vi "SHI_Cryopump_interface.vi"() -> ()   [LabVIEW 2017]
uses:
  Type_Defs/Cryo_Pump_MCC_Status.ctl
  Type_Defs/Cryo_Pump_MCC_CryoPump.ctl
  Type_Defs/Cryo_Pump_MCC_RoughingInterlock.ctl
  Type_Defs/Cryo_Pump_MCC_Status_Status.ctl
  Type_Defs/Cryo_Pump_MCC_Start_Regen.ctl
  Type_Defs/Cryo_Pump_MCC_First_Stage_Temp_CTL.ctl
  Type_Defs/Cryo_Pump_MCC_Params_Power_Failure_Recovery.ctl
  Type_Defs/Cryo_Pump_MCC_Regen_Params.ctl
  Type_Defs/Cryo_Pump_Compressor_Status.ctl
  Type_Defs/Cryo_Pump_Compressor_Status_Status.ctl
  <vilib>/httpClient/ClientHandle.ctl
  Type_Defs/Cryo_Pump_Plots.ctl
  Type_Defs/Cryo_Pump_MCC_Params.ctl
  msg7171_linux.llb/send single message.vi
  msg7171_linux.llb/send multiple messages.vi
  <vilib>/httpClient/POSTBuffer.vi
  <vilib>/httpClient/LabVIEWHTTPClient.lvlib
panel:
  in  "Cold Head Start":bool
  in  "Compressor On":bool
  in  "Roughing_Ilock_Permission":bool
  in  "TC_Pressure_Guage":bool
  in  "Roughing Valve":bool
  in  "Purge Valve":bool
  in  "Send Regen Start":bool
  out "Compressor":T1
  in  "2nd Stage Temp CTL":u32 max=320 step=1
  out "Regen Time":u32
  out "Regen Step Timer":u32
  in  "Regen Start Delay":u32 max=59994 step=1
  in  "Regen Parameters":T3 {"z" max=1 step=1; "G" max=9999 step=1; "C" min=1 max=3 step=1; "A" max=1 step=1; "6" max=80 step=1; "5" max=200 step=1; "4" min=1 max=100 step=1; "3" min=25 max=200 step=1; "2" max=200 step=1; "1" max=9990 step=1; "0" max=59994 step=1}
  out "Regen Cycles":u32
  out "Power Failure Recovery Status":string
  in  "Power Failure Recovery":T4 items=["Disabled", "Enabled", "Enabled only when Stage 2 < Restart Temp."]
  out "MCC Version":string
  out "Last Rate Of Rise Value":u32
  in  "1st Stage Temp Ctl":T5 {"method" items=["ExtHeat", "1st s ctl", "2nd sctl", "Dual"]; "temp" max=320 step=1}
  out "Failed Repurge Cycles":u32
  out "Failed Rate Of Rise Cycles":u32
  out "Elapsed Time":u32
  in  "Start Regen Parameter":T6=enum."Start full regeneration cycle"
  out "MCC Status":T7
  out "Get Params json":string
  out "Get Status json":string
  in  "exit":bool
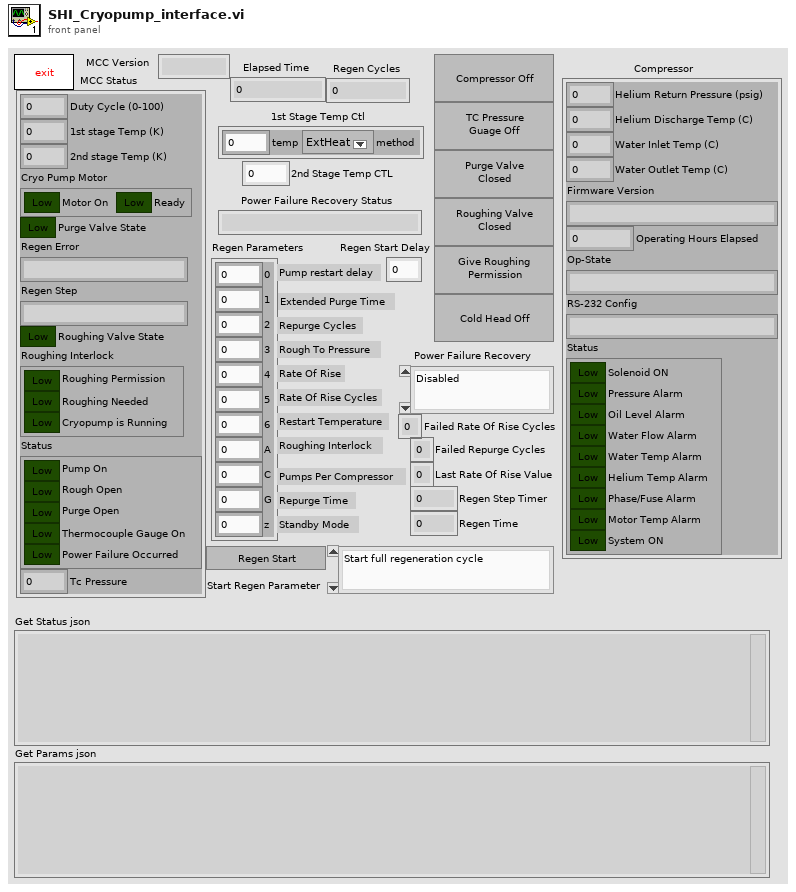
[diagram p1: front panel]
types:
  T1 = typedef "Cryo_Pump_Compressor_Status.ctl" = cluster{"Helium Return Pressure (psig)":u32, "Helium Discharge Temp (C)":u32, "Water Inlet Temp (C)":u32, "Water Outlet Temp (C)":u32, "Firmware Version":string, "Operating Hours Elapsed":dbl, "Op-State":string, "RS-232 Config":string, "Status":T2}
  T2 = typedef "Cryo_Pump_Compressor_Status_Status.ctl" = cluster{"Solenoid ON":bool, "Pressure Alarm":bool, "Oil Level Alarm":bool, "Water Flow Alarm":bool, "Water Temp Alarm":bool, "Helium Temp Alarm":bool, "Phase/Fuse Alarm":bool, "Motor Temp Alarm":bool, "System ON":bool}
  T3 = typedef "Cryo_Pump_MCC_Regen_Params.ctl" = cluster{"0":u32, "1":u32, "2":u32, "3":u32, "4":u32, "5":u32, "6":u32, "A":u32, "C":u32, "G":u32, "z":u32}
  T4 = typedef "Cryo_Pump_MCC_Params_Power_Failure_Recovery.ctl" = u16
  T5 = typedef "Cryo_Pump_MCC_First_Stage_Temp_CTL.ctl" = cluster{"temp":u32, "method":u32}
  T6 = typedef "Cryo_Pump_MCC_Start_Regen.ctl" = enum16{"Abort current regeneration cycle", "Start full regeneration cycle", "Start fast regeneration cycle", "Activate stand-by pump module for normal pumping operation", "Warm up cryopump and stop"}
  T7 = typedef "Cryo_Pump_MCC_Status.ctl" = cluster{"Duty Cycle (0-100)":dbl, "1st stage Temp (K)":dbl, "2nd stage Temp (K)":dbl, "Cryo Pump Motor":T8, "Purge Valve State":bool, "Regen Error":string, "Regen Step":string, "Roughing Valve State":bool, "Roughing Interlock":T9, "Status":T10, "Tc Pressure":dbl}
  T8 = typedef "Cryo_Pump_MCC_CryoPump.ctl" = cluster{"Motor On":bool, "Ready":bool}
  T9 = typedef "Cryo_Pump_MCC_RoughingInterlock.ctl" = cluster{"Roughing Permission":bool, "Roughing Needed":bool, "Cryopump is Running":bool}
  T10 = typedef "Cryo_Pump_MCC_Status_Status.ctl" = cluster{"Pump On":bool, "Rough Open":bool, "Purge Open":bool, "Thermocouple Gauge On":bool, "Power Failure Occurred":bool}
  T11 = typedef "Cryo_Pump_Plots.ctl" = cluster{"Duty Cycle (0-100)":dbl, "1st stage Temp (K)":dbl, "2nd stage Temp (K)":dbl, "Helium Return Pressure (psig)":u32, "Helium Discharge Temp (C)":u32, "Water Inlet Temp (C)":u32, "Water Outlet Temp (C)":u32}
  T12 = typedef "LabVIEWHTTPClient.lvlib/ClientHandle.ctl" = refnum<k1>
  T13 = cluster{"go":bool, "Http session":T12, "URL prefex":string, "Next get param":u32}
  T14 = typedef "Cryo_Pump_MCC_Params.ctl" = cluster{"MCC Version":string, "First Stage Temp CTL":T5, "Second Stage Temp CTL":u32, "Tc Pressure State":bool, "Elapsed Time":u32, "Power Failure Recovery":T4, "Power Failure Recovery Status":string, "Regen Time":u32, "Regen Parameters":T3, "Regen Start Delay":u32, "Regen Step Timer":u32, "Failed Rate Of Rise Cycles":u32, "Failed Repurge Cycles":u32, "Last Rate Of Rise Value":u32, "Regen Cycles":u32}
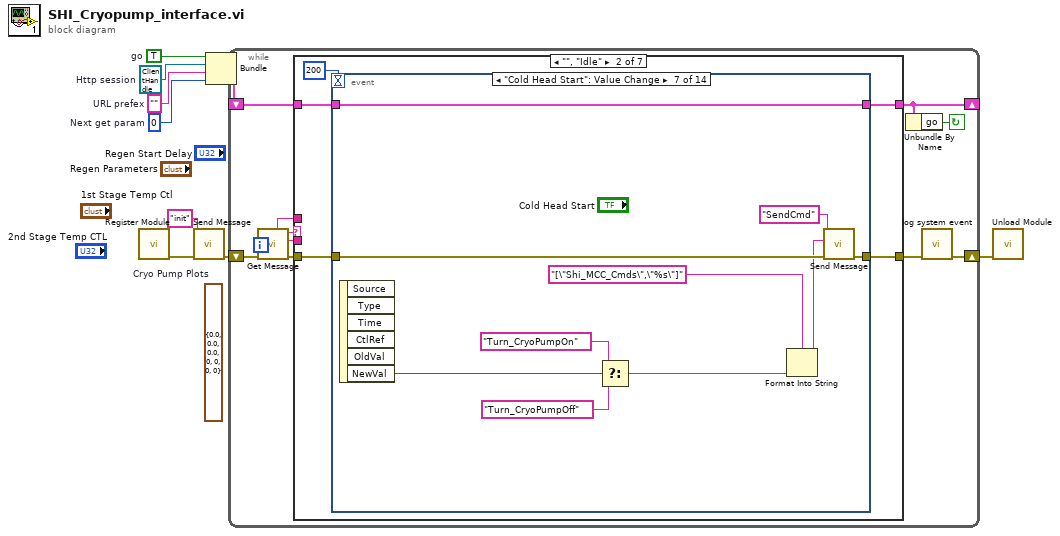
[diagram p0: block diagram]
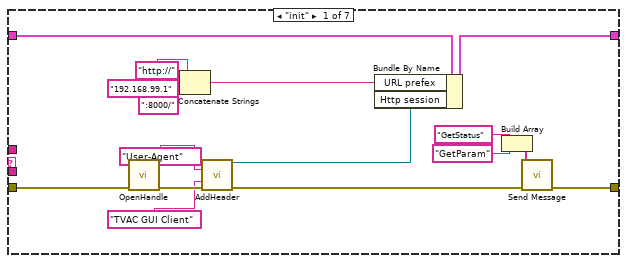
[diagram p2: hidden frame]
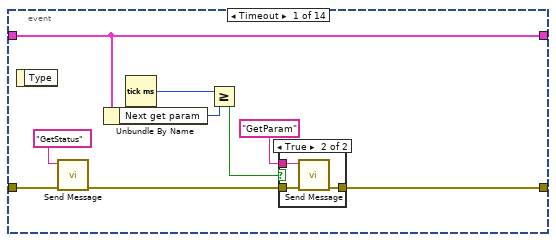
[diagram p3: hidden frame]
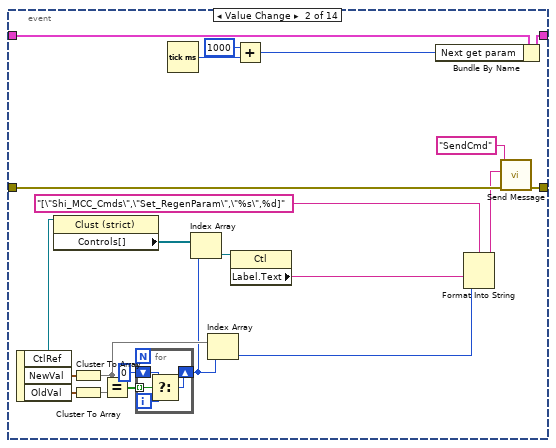
[diagram p5: hidden frame]
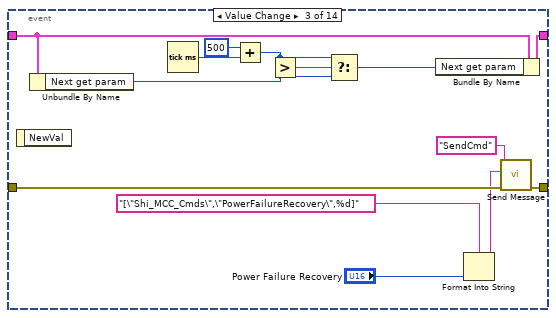
[diagram p6: hidden frame]
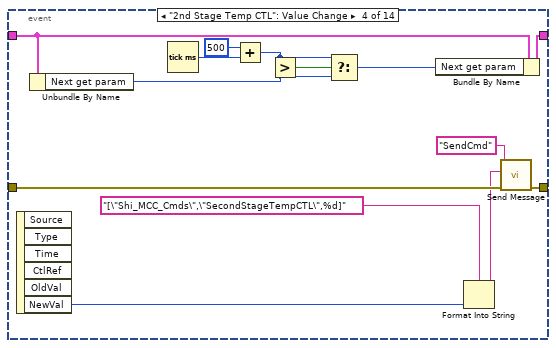
[diagram p7: hidden frame]
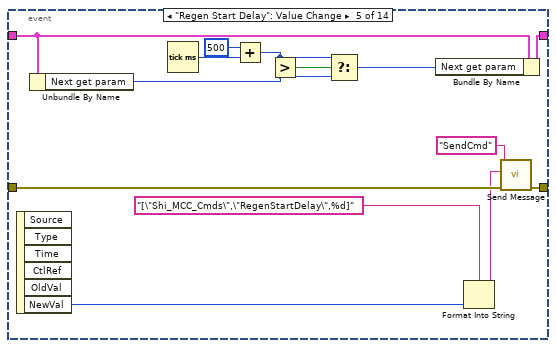
[diagram p8: hidden frame]
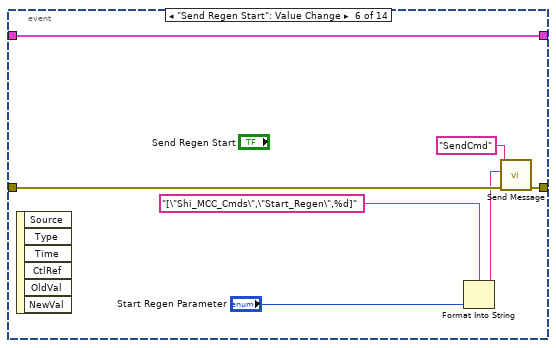
[diagram p9: hidden frame]
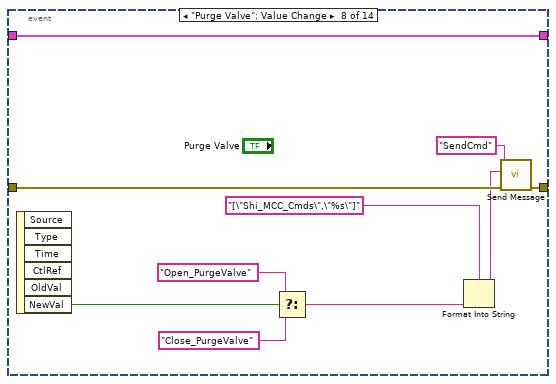
[diagram p10: hidden frame]
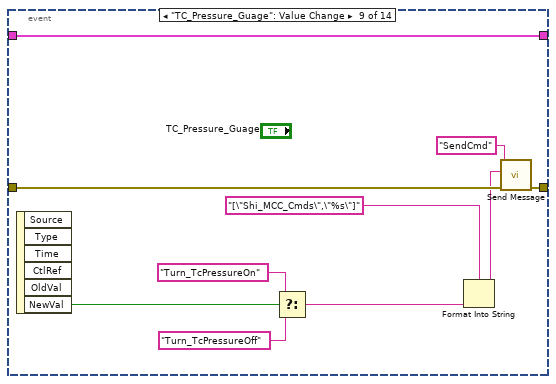
[diagram p11: hidden frame]
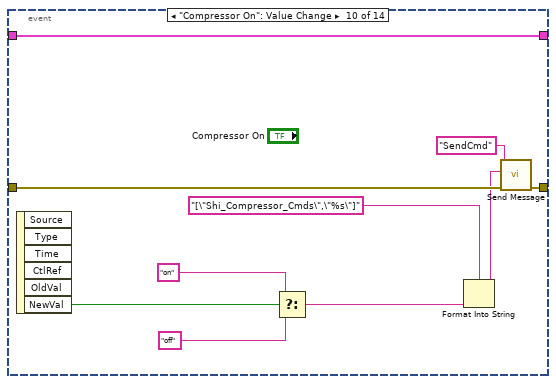
[diagram p12: hidden frame]
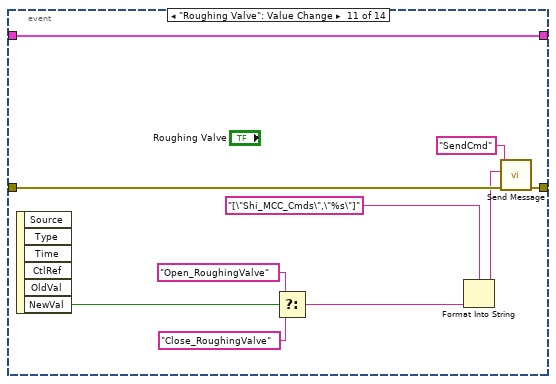
[diagram p13: hidden frame]
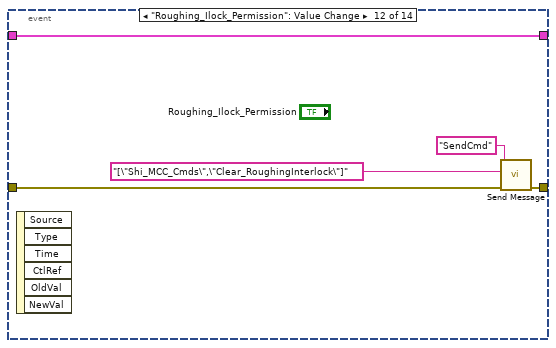
[diagram p14: hidden frame]
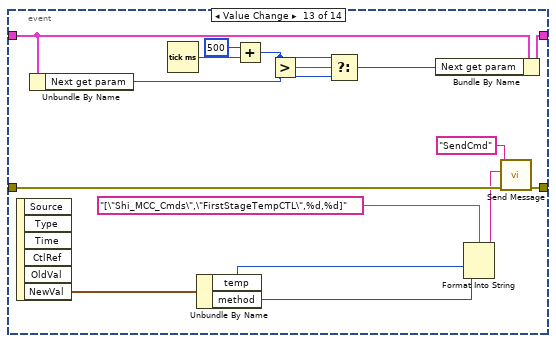
[diagram p15: hidden frame]
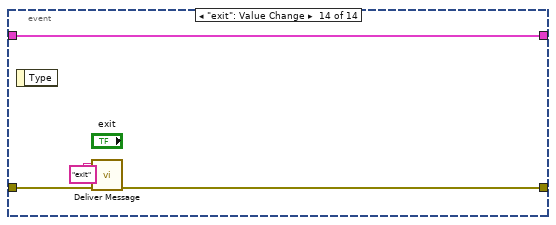
[diagram p16: hidden frame]
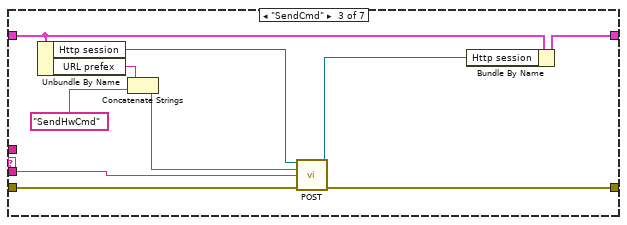
[diagram p17: hidden frame]
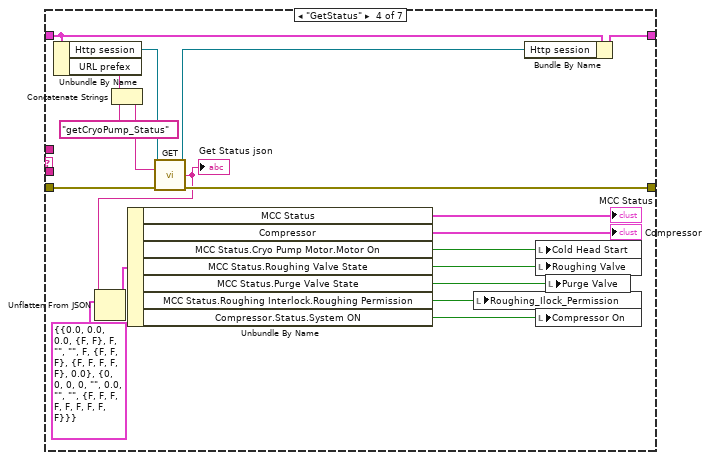
[diagram p18: hidden frame]
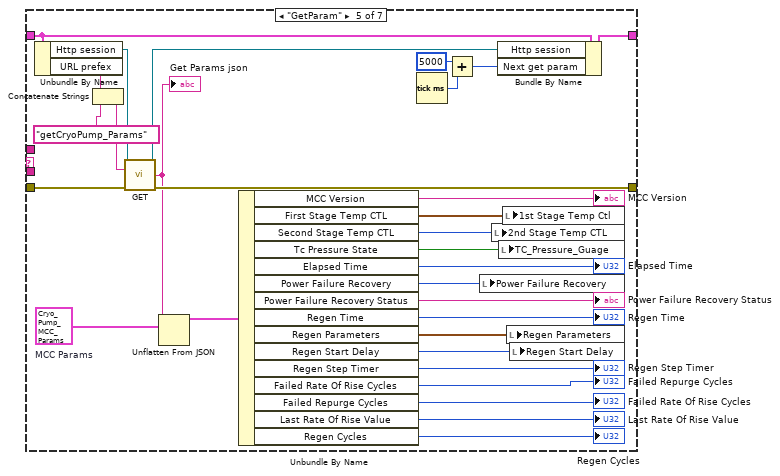
[diagram p19: hidden frame]
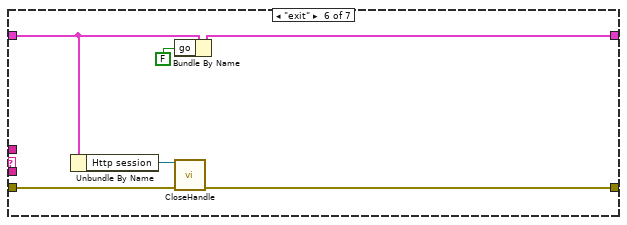
[diagram p20: hidden frame]
diagram:
  (unwired) T11 {"Duty Cycle (0-100)"=0.0, "1st stage Temp (K)"=0.0, "2nd stage Temp (K)"=0.0, "Helium Return Pressure (psig)"=0, "Helium Discharge Temp (C)"=0, "Water Inlet Temp (C)"=0, "Water Outlet Temp (C)"=0}  # Cryo Pump Plots
  w1 = u32 0  # Next get param
  w5 = ""  # URL prefex
  w6 = T12 refnum  # Http session
  w7 = TRUE  # go
  n1 = call "Register Module.vi"() -> ("error out"=w3:errorcluster)  [unwired: 10 in, 1 out]
  n2 = call-poly "Send Message.vi"("error in (no error)"=w3, "event"="init") -> ("error out"=w2:errorcluster)  [unwired: 9 in]
  n3 = Bundle("go"=w7, "Http session"=w6, "URL prefex"=w5, "Next get param"=w1) -> (w9:T13)  [unwired: 1 in]
  n4 = while {
    shift-left: w9 -> [w16]
    shift-right: [w13] -> _
    shift-right: [w11] -> w8
    shift-left: w2 -> [w19]
    stop <- w12 continue-if-true
    n5 = call "Get Message.vi"("error in (no error)"=w19) -> ("error out"=w17:errorcluster, "event buffer"=w18:string, "event"=w15:string, "source"=w14:string)  [unwired: 7 in]
    n6 = case shown="\"\", \"Idle\"" w15 {
      selector: w15 -> [_ _ _ _ _ _ w272]
      tunnel: [w27 w38 w209 w226 w256 w269 w274] -> w13
      tunnel: w16 -> [w36 w37 w208 w225 w255 w264 w274]
      tunnel: w18 -> [_ _ w205 _ _ _ _]
      tunnel: w17 -> [w31 w39 w207 w228 w258 w267 w273]
      tunnel: w14 -> [_ _ _ _ _ _ w271]
      tunnel: [w23 w41 w206 w227 w257 w266 w270] -> w10
      frame "init" {
        n7 = call <vilib>:"OpenHandle.vi"("error in (no error)"=w31) -> ("client handle out"=w32:T12, "error out"=w35:errorcluster)  [unwired: 13 in]
        n8 = Concatenate Strings("http://" ("url"), "192.168.99.1" ("Address"), ":8000/" ("url")) -> (w26:string)
        n9 = call <vilib>:"AddHeader.vi"("client handle"=w32, "header"="User-Agent", "value"="TVAC GUI Client", "error in (no error)"=w35) -> ("client handle out"=w25:T12, "error out"=w24:errorcluster)  [unwired: 10 in]
        n10 = Bundle By Name(cluster=w36, "URL prefex"=w26, "Http session"=w25) -> (w27:T13)
        n11 = Build Array("GetStatus" ("event"), "GetParam" ("event")) -> (w21:string[])
        n12 = call-poly "Send Message.vi"("error in (no error)"=w24, "event"=w21) -> ("error out"=w23:errorcluster)  [unwired: 9 in]
      }
      frame "", "Idle" {
        n13 = event shown="[6] \"Cold Head Start\": Value Change" {
          selector: _ -> [_ _ _ _ _ _ _ _ _ _ _ _ _ _]
          dyn-events: _ -> [_ _ _ _ _ _ _ _ _ _ _ _ _ _]
          timeout: 200 ("milliseconds to wait") -> [_ _ _ _ _ _ _ _ _ _ _ _ _ _]
          tunnel: w39 -> [w50 w72 w94 w108 w122 w129 w139 w149 w159 w169 w179 w184 w200 w204]
          tunnel: [w46 w71 w93 w107 w121 w128 w138 w148 w158 w168 w178 w183 w199 w203] -> w41
          tunnel: [w42 w58 w88 w102 w116 w123 w130 w140 w150 w160 w170 w180 w194 w201] -> w38
          tunnel: w37 -> [w42 w59 w89 w103 w117 w123 w130 w140 w150 w160 w170 w180 w195 w201]
          event Timeout {
            n14 = event-data() -> ()  [unwired: 1 in, 1 out]
            n15 = call-poly "Send Message.vi"("error in (no error)"=w50, "event"="GetStatus") -> ("error out"=w48:errorcluster)  [unwired: 9 in]
            n16 = Unbundle By Name(w42) -> ("Next get param"=w43:u32)
            n17 = Tick Count (ms)() -> (millisecond timer value=w45:u32)
            n18 = Greater Or Equal?(x=w45, y=w43) -> (x >= y?=w44:bool)
            n19 = case shown="True" w44 {
              tunnel: w48 -> [w51 w54]
              tunnel: [w51 w53] -> w46
              tunnel: "GetParam" ("event") -> [_ w52]
              frame False {
              }
              frame True {
                n20 = call-poly "Send Message.vi"("error in (no error)"=w54, "event"=w52) -> ("error out"=w53:errorcluster)  [unwired: 9 in]
              }
            }
          }
          event Value Change {
            n21 = event-data() -> ("CtlRef"=w63:refnum<vi>, "NewVal"=w73:T3, "OldVal"=w76:T3)  [unwired: 1 in]
            n22 = property class="Clust (strict)"(reference=w63) -> ("Controls[]"=w68:refnum<vi>[])  [unwired: 1 in, 2 out]
            n23 = Cluster To Array(cluster=w73) -> (array=w69:u32[])
            n24 = Cluster To Array(cluster=w76) -> (array=w70:u32[])
            n25 = Equal?(x=w69, y=w70) -> (x = y?=w75:bool[])
            n26 = for {
              tunnel: w75 -> [w80] mode=indexing
              shift-right: [w79] -> w67
              shift-left: 0 -> [w78]
              i -> [w77]
              n27 = Select(t=w78, s=w80, f=w77) -> (s? t:f=w79:i32)
            }
            n28 = Tick Count (ms)() -> (millisecond timer value=w57:u32)
            n29 = Index Array(array=w68, index=w67) -> (element=w66:refnum<vi>)
            n30 = Index Array(array=w69, index=w67) -> (element=w61:u32)
            n31 = property class="Ctl"(reference=w66) -> ("Label.Text"=w60:string)  [unwired: 1 in, 2 out]
            n32 = Add(x=u32 1000, y=w57) -> (x+y=w55:u32)
            n33 = Bundle By Name(cluster=w59, "Next get param"=w55) -> (w58:T13)
            n34 = Format Into String(format string="[\"Shi_MCC_Cmds\",\"Set_RegenParam\",\"%s\",%d]" ("string"), w60, w61) -> (resulting string=w62:string)  [unwired: 2 in, 1 out]
            n35 = call-poly "Send Message.vi"("error in (no error)"=w72, "event buffer"=w62, "event"="SendCmd") -> ("error out"=w71:errorcluster)  [unwired: 8 in]
          }
          event Value Change {
            n36 = event-data() -> ()  [unwired: 1 in, 1 out]
            n37 = Unbundle By Name(w89) -> ("Next get param"=w83:u32)
            n38 = Tick Count (ms)() -> (millisecond timer value=w87:u32)
            n39 = Add(x=u32 500, y=w87) -> (x+y=w82:u32)
            n40 = Greater?(x=w82, y=w83) -> (0:w85:bool)
            n41 = Select(t=w82, s=w85, f=w83) -> (s? t:f=w84:u32)
            n42 = Bundle By Name(cluster=w89, "Next get param"=w84) -> (w88:T13)
            n43 = Format Into String(format string="[\"Shi_MCC_Cmds\",\"PowerFailureRecovery\",%d]" ("string"), "Power Failure Recovery") -> (resulting string=w90:string)  [unwired: 2 in, 1 out]
            n44 = call-poly "Send Message.vi"("error in (no error)"=w94, "event buffer"=w90, "event"="SendCmd") -> ("error out"=w93:errorcluster)  [unwired: 8 in]
          }
          event "2nd Stage Temp CTL": Value Change {
            n45 = event-data() -> ("NewVal"=w95:u32)  [unwired: 1 in, 5 out]
            n46 = Unbundle By Name(w103) -> ("Next get param"=w97:u32)
            n47 = Tick Count (ms)() -> (millisecond timer value=w101:u32)
            n48 = Add(x=u32 500, y=w101) -> (x+y=w96:u32)
            n49 = Greater?(x=w96, y=w97) -> (0:w99:bool)
            n50 = Select(t=w96, s=w99, f=w97) -> (s? t:f=w98:u32)
            n51 = Bundle By Name(cluster=w103, "Next get param"=w98) -> (w102:T13)
            n52 = Format Into String(format string="[\"Shi_MCC_Cmds\",\"SecondStageTempCTL\",%d]" ("string"), w95) -> (resulting string=w104:string)  [unwired: 2 in, 1 out]
            n53 = call-poly "Send Message.vi"("error in (no error)"=w108, "event buffer"=w104, "event"="SendCmd") -> ("error out"=w107:errorcluster)  [unwired: 8 in]
          }
          event "Regen Start Delay": Value Change {
            n54 = event-data() -> ("NewVal"=w109:u32)  [unwired: 1 in, 5 out]
            n55 = Unbundle By Name(w117) -> ("Next get param"=w111:u32)
            n56 = Tick Count (ms)() -> (millisecond timer value=w115:u32)
            n57 = Add(x=u32 500, y=w115) -> (x+y=w110:u32)
            n58 = Greater?(x=w110, y=w111) -> (0:w113:bool)
            n59 = Select(t=w110, s=w113, f=w111) -> (s? t:f=w112:u32)
            n60 = Bundle By Name(cluster=w117, "Next get param"=w112) -> (w116:T13)
            n61 = Format Into String(format string="[\"Shi_MCC_Cmds\",\"RegenStartDelay\",%d]" ("string"), w109) -> (resulting string=w118:string)  [unwired: 2 in, 1 out]
            n62 = call-poly "Send Message.vi"("error in (no error)"=w122, "event buffer"=w118, "event"="SendCmd") -> ("error out"=w121:errorcluster)  [unwired: 8 in]
          }
          event "Send Regen Start": Value Change {
            n63 = event-data() -> ()  [unwired: 1 in, 6 out]
            n64 = Format Into String(format string="[\"Shi_MCC_Cmds\",\"Start_Regen\",%d]" ("string"), "Start Regen Parameter") -> (resulting string=w125:string)  [unwired: 2 in, 1 out]
            n65 = call-poly "Send Message.vi"("error in (no error)"=w129, "event buffer"=w125, "event"="SendCmd") -> ("error out"=w128:errorcluster)  [unwired: 8 in]
          }
          event "Cold Head Start": Value Change {
            n66 = event-data() -> ("NewVal"=w134:bool)  [unwired: 1 in, 5 out]
            n67 = Select(t="Turn_CryoPumpOn", s=w134, f="Turn_CryoPumpOff") -> (s? t:f=w133:string)
            n68 = Format Into String(format string="[\"Shi_MCC_Cmds\",\"%s\"]" ("string"), w133) -> (resulting string=w135:string)  [unwired: 2 in, 1 out]
            n69 = call-poly "Send Message.vi"("error in (no error)"=w139, "event buffer"=w135, "event"="SendCmd") -> ("error out"=w138:errorcluster)  [unwired: 8 in]
          }
          event "Purge Valve": Value Change {
            n70 = event-data() -> ("NewVal"=w144:bool)  [unwired: 1 in, 5 out]
            n71 = Select(t="Open_PurgeValve", s=w144, f="Close_PurgeValve") -> (s? t:f=w143:string)
            n72 = Format Into String(format string="[\"Shi_MCC_Cmds\",\"%s\"]" ("string"), w143) -> (resulting string=w145:string)  [unwired: 2 in, 1 out]
            n73 = call-poly "Send Message.vi"("error in (no error)"=w149, "event buffer"=w145, "event"="SendCmd") -> ("error out"=w148:errorcluster)  [unwired: 8 in]
          }
          event "TC_Pressure_Guage": Value Change {
            n74 = event-data() -> ("NewVal"=w154:bool)  [unwired: 1 in, 5 out]
            n75 = Select(t="Turn_TcPressureOn", s=w154, f="Turn_TcPressureOff") -> (s? t:f=w153:string)
            n76 = Format Into String(format string="[\"Shi_MCC_Cmds\",\"%s\"]" ("string"), w153) -> (resulting string=w155:string)  [unwired: 2 in, 1 out]
            n77 = call-poly "Send Message.vi"("error in (no error)"=w159, "event buffer"=w155, "event"="SendCmd") -> ("error out"=w158:errorcluster)  [unwired: 8 in]
          }
          event "Compressor On": Value Change {
            n78 = event-data() -> ("NewVal"=w164:bool)  [unwired: 1 in, 5 out]
            n79 = Select(t="on", s=w164, f="off") -> (s? t:f=w163:string)
            n80 = Format Into String(format string="[\"Shi_Compressor_Cmds\",\"%s\"]" ("string"), w163) -> (resulting string=w165:string)  [unwired: 2 in, 1 out]
            n81 = call-poly "Send Message.vi"("error in (no error)"=w169, "event buffer"=w165, "event"="SendCmd") -> ("error out"=w168:errorcluster)  [unwired: 8 in]
          }
          event "Roughing Valve": Value Change {
            n82 = event-data() -> ("NewVal"=w174:bool)  [unwired: 1 in, 5 out]
            n83 = Select(t="Open_RoughingValve", s=w174, f="Close_RoughingValve") -> (s? t:f=w173:string)
            n84 = Format Into String(format string="[\"Shi_MCC_Cmds\",\"%s\"]" ("string"), w173) -> (resulting string=w175:string)  [unwired: 2 in, 1 out]
            n85 = call-poly "Send Message.vi"("error in (no error)"=w179, "event buffer"=w175, "event"="SendCmd") -> ("error out"=w178:errorcluster)  [unwired: 8 in]
          }
          event "Roughing_Ilock_Permission": Value Change {
            n86 = event-data() -> ()  [unwired: 1 in, 6 out]
            n87 = call-poly "Send Message.vi"("error in (no error)"=w184, "event buffer"="[\"Shi_MCC_Cmds\",\"Clear_RoughingInterlock\"]" ("string"), "event"="SendCmd") -> ("error out"=w183:errorcluster)  [unwired: 8 in]
          }
          event Value Change {
            n88 = event-data() -> ("NewVal"=w185:T5)  [unwired: 1 in, 5 out]
            n89 = Unbundle By Name(w195) -> ("Next get param"=w189:u32)
            n90 = Tick Count (ms)() -> (millisecond timer value=w193:u32)
            n91 = Unbundle By Name(w185) -> ("temp"=w187:u32, "method"=w186:u32)
            n92 = Add(x=u32 500, y=w193) -> (x+y=w188:u32)
            n93 = Greater?(x=w188, y=w189) -> (0:w191:bool)
            n94 = Select(t=w188, s=w191, f=w189) -> (s? t:f=w190:u32)
            n95 = Bundle By Name(cluster=w195, "Next get param"=w190) -> (w194:T13)
            n96 = Format Into String(format string="[\"Shi_MCC_Cmds\",\"FirstStageTempCTL\",%d,%d]" ("string"), w187, w186) -> (resulting string=w196:string)  [unwired: 2 in, 1 out]
            n97 = call-poly "Send Message.vi"("error in (no error)"=w200, "event buffer"=w196, "event"="SendCmd") -> ("error out"=w199:errorcluster)  [unwired: 8 in]
          }
          event "exit": Value Change {
            n98 = event-data() -> ()  [unwired: 1 in, 1 out]
            n99 = call "Deliver Message.vi"("error in (no error)"=w204, "event"="exit") -> ("error out"=w203:errorcluster)  [unwired: 9 in]
          }
        }
      }
      frame "SendCmd" {
        n100 = Unbundle By Name(w208) -> ("Http session"=w213:T12, "URL prefex"=w211:string)
        n101 = Concatenate Strings(w211, "SendHwCmd" ("url")) -> (w212:string)
        n102 = call-poly <vilib>:"POST.vi"("client handle"=w213, "url"=w212, "buffer"=w205, "error in (no error)"=w207) -> ("client handle out"=w214:T12, "error out"=w206:errorcluster)  [unwired: 8 in, 2 out]
        n103 = Bundle By Name(cluster=w208, "Http session"=w214) -> (w209:T13)
      }
      frame "GetStatus" {
        n104 = Unbundle By Name(w225) -> ("Http session"=w232:T12, "URL prefex"=w230:string)
        n105 = Concatenate Strings(w230, "getCryoPump_Status" ("url")) -> (w231:string)
        n106 = call <vilib>:"GET.vi"("client handle"=w232, "url"=w231, "error in (no error)"=w228) -> ("client handle out"=w233:T12, "body"=w215:string, "error out"=w227:errorcluster)  [unwired: 9 in, 1 out]
        "Get Status json" <- w215
        n107 = Unflatten From JSON(JSON string=w215, type and defaults=cluster{"MCC Status":T7, "Compressor":T1} {"MCC Status"={"Duty Cycle (0-100)"=0.0, "1st stage Temp (K)"=0.0, "2nd stage Temp (K)"=0.0, "Cryo Pump Motor"={"Motor On"=FALSE, "Ready"=FALSE}, "Purge Valve State"=FALSE, "Regen Error"="", "Regen Step"="", "Roughing Valve State"=FALSE, "Roughing Interlock"={"Roughing Permission"=FALSE, "Roughing Needed"=FALSE, "Cryopump is Running"=FALSE}, "Status"={"Pump On"=FALSE, "Rough Open"=FALSE, "Purge Open"=FALSE, "Thermocouple Gauge On"=FALSE, "Power Failure Occurred"=FALSE}, "Tc Pressure"=0.0}, "Compressor"={"Helium Return Pressure (psig)"=0, "Helium Discharge Temp (C)"=0, "Water Inlet Temp (C)"=0, "Water Outlet Temp (C)"=0, "Firmware Version"="", "Operating Hours Elapsed"=0.0, "Op-State"="", "RS-232 Config"="", "Status"={"Solenoid ON"=FALSE, "Pressure Alarm"=FALSE, "Oil Level Alarm"=FALSE, "Water Flow Alarm"=FALSE, "Water Temp Alarm"=FALSE, "Helium Temp Alarm"=FALSE, "Phase/Fuse Alarm"=FALSE, "Motor Temp Alarm"=FALSE, "System ON"=FALSE}}}) -> (value=w224:cluster{"MCC Status":T7, "Compressor":T1})  [unwired: 5 in, 1 out]
        n108 = Unbundle By Name(w224) -> ("MCC Status"=→"MCC Status":T7, "Compressor"=→"Compressor":T1, "MCC Status.Cryo Pump Motor.Motor On"=w222:bool, "MCC Status.Roughing Valve State"=w221:bool, "MCC Status.Purge Valve State"=w220:bool, "MCC Status.Roughing Interlock.Roughing Permission"=w219:bool, "Compressor.Status.System ON"=w218:bool)
        n109 = local write "Roughing_Ilock_Permission"(w219) -> ()
        n110 = Bundle By Name(cluster=w225, "Http session"=w233) -> (w226:T13)
        n111 = local write "Cold Head Start"(w222) -> ()
        n112 = local write "Roughing Valve"(w221) -> ()
        n113 = local write "Compressor On"(w218) -> ()
        n114 = local write "Purge Valve"(w220) -> ()
      }
      frame "GetParam" {
        w249 = T14 {"MCC Version"="", "First Stage Temp CTL"={"temp"=0, "method"=0}, "Second Stage Temp CTL"=0, "Tc Pressure State"=FALSE, "Elapsed Time"=0, "Power Failure Recovery"=0, "Power Failure Recovery Status"="", "Regen Time"=0, "Regen Parameters"={"0"=0, "1"=0, "2"=0, "3"=0, "4"=0, "5"=0, "6"=0, "A"=0, "C"=0, "G"=0, "z"=0}, "Regen Start Delay"=0, "Regen Step Timer"=0, "Failed Rate Of Rise Cycles"=0, "Failed Repurge Cycles"=0, "Last Rate Of Rise Value"=0, "Regen Cycles"=0}  # MCC Params
        n115 = Unbundle By Name(w255) -> ("Http session"=w262:T12, "URL prefex"=w260:string)
        n116 = Concatenate Strings(w260, "getCryoPump_Params" ("url")) -> (w261:string)
        n117 = call <vilib>:"GET.vi"("client handle"=w262, "url"=w261, "error in (no error)"=w258) -> ("client handle out"=w263:T12, "body"=w250:string, "error out"=w257:errorcluster)  [unwired: 9 in, 1 out]
        "Get Params json" <- w250
        n118 = Unflatten From JSON(JSON string=w250, type and defaults=w249) -> (value=w254:T14)  [unwired: 5 in, 1 out]
        n119 = Unbundle By Name(w254) -> ("MCC Version"=→"MCC Version":string, "First Stage Temp CTL"=w247:T5, "Second Stage Temp CTL"=w248:u32, "Tc Pressure State"=w246:bool, "Elapsed Time"=→"Elapsed Time":u32, "Power Failure Recovery"=w243:T4, "Power Failure Recovery Status"=→"Power Failure Recovery Status":string, "Regen Time"=→"Regen Time":u32, "Regen Parameters"=w244:T3, "Regen Start Delay"=w245:u32, "Regen Step Timer"=→"Regen Step Timer":u32, "Failed Rate Of Rise Cycles"=→"Failed Repurge Cycles":u32, "Failed Repurge Cycles"=→"Failed Rate Of Rise Cycles":u32, "Last Rate Of Rise Value"=→"Last Rate Of Rise Value":u32, "Regen Cycles"=→"Regen Cycles":u32)
        n120 = Tick Count (ms)() -> (millisecond timer value=w253:u32)
        n121 = Add(x=u32 5000, y=w253) -> (x+y=w251:u32)
        n122 = local write "Power Failure Recovery"(w243) -> ()
        n123 = local write "2nd Stage Temp CTL"(w248) -> ()
        n124 = Bundle By Name(cluster=w255, "Http session"=w263, "Next get param"=w251) -> (w256:T13)
        n125 = local write "TC_Pressure_Guage"(w246) -> ()
        n126 = local write "1st Stage Temp Ctl"(w247) -> ()
        n127 = local write "Regen Parameters"(w244) -> ()
        n128 = local write "Regen Start Delay"(w245) -> ()
      }
      frame "exit" {
        n129 = Unbundle By Name(w264) -> ("Http session"=w265:T12)
        n130 = Bundle By Name(cluster=w264, "go"=FALSE ("Bundle Element")) -> (w269:T13)
        n131 = call <vilib>:"CloseHandle.vi"("client handle"=w265, "error in (no error)"=w267) -> ("error out"=w266:errorcluster)  [unwired: 13 in]
      }
      frame Default {
        n132 = call "Unknown Message Dialog.vi"("source"=w271, "error in (no error)"=w273, "event name"=w272) -> ("error out"=w270:errorcluster)  [unwired: 8 in]
      }
    }
    n133 = Unbundle By Name(w13) -> ("go"=w12:bool)
    n134 = call "log system event.vi"("error in (no error)"=w10) -> ("error out"=w11:errorcluster)  [unwired: 9 in, 1 out]
  }
  n135 = call "Unload Module.vi"("error in (no error)"=w8) -> ()  [unwired: 10 in, 1 out]
